vi "SubVI Tester.vi"() -> ()   [LabVIEW 2012]
uses:
  weather data.ctl
panel:
  in  "Max Windspeed":dbl
  in  "Current Windspeed":dbl
  in  "Weather Data In":T1={"Current Temperature"=0.0, "Max Temperature"=0.0, "Min Temperature"=0.0, "Warning Text"="", "Warning?"=FALSE, "Enum"=enum."Fahrenheit", "Current Windspeed"=0.0, "Max Windspeed"=0.0, "Windspeed Warning?"=FALSE, "Windspeed Warning Text"="No Warning"}
  out "Weather Data out":T1={"Current Temperature"=0.0, "Max Temperature"=0.0, "Min Temperature"=0.0, "Warning Text"="", "Warning?"=FALSE, "Enum"=enum."Fahrenheit", "Current Windspeed"=0.0, "Max Windspeed"=0.0, "Windspeed Warning?"=FALSE, "Windspeed Warning Text"="No Warning"}
  in  "Min Temperature":dbl=10.0
  in  "Max Temperature":dbl=30.0
  in  "Stop":bool
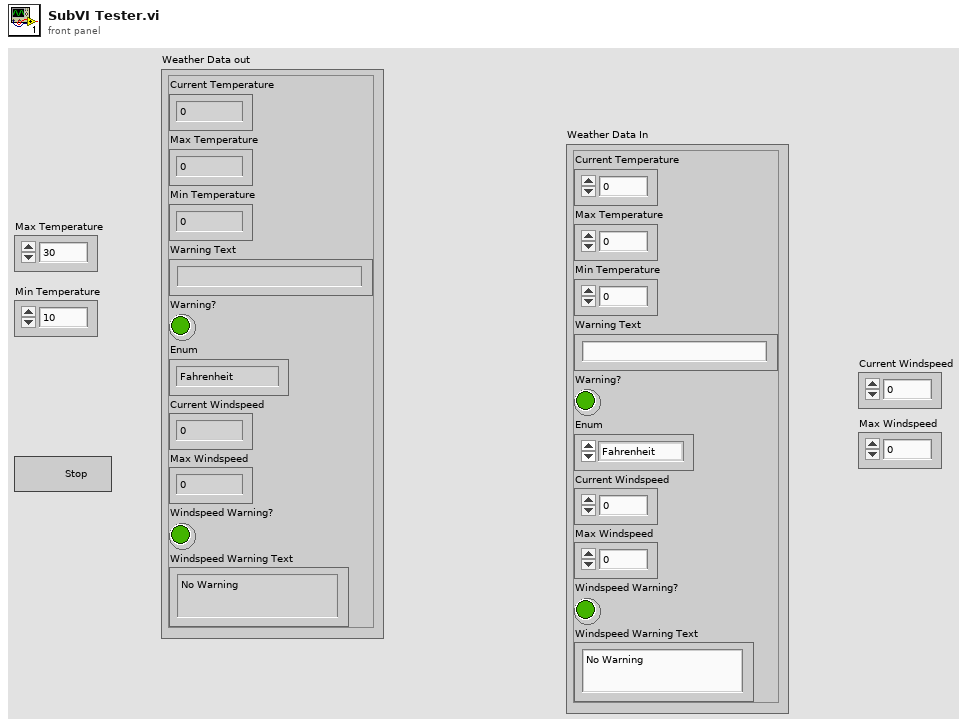
[diagram p1: front panel]
types:
  T1 = typedef "weather data.ctl" = cluster{"Current Temperature":dbl, "Max Temperature":dbl, "Min Temperature":dbl, "Warning Text":string, "Warning?":bool, "Enum":enum16{"Fahrenheit", "Celcius"}, "Current Windspeed":dbl, "Max Windspeed":dbl, "Windspeed Warning?":bool, "Windspeed Warning Text":string}
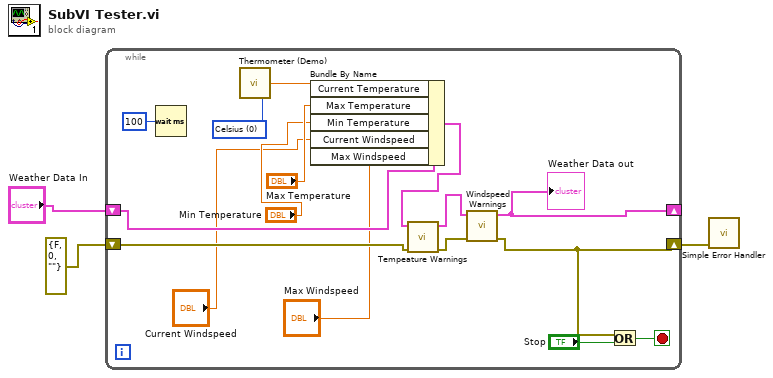
[diagram p0: block diagram]
diagram:
  n1 = while {
    shift-right: [w9] -> w3
    shift-left: errorcluster {"status"=FALSE, "code"=0, "source"=""} ("error in") -> [w16]
    shift-right: [w6] -> _
    shift-left: "Weather Data In" -> [w12]
    stop <- w17 stop-if-true
    w10 = u16 0 items=["Celsius", "Fahrenheit"] ("Units (0: Celsius)")
    n2 = Wait (ms)(milliseconds to wait=u32 100) -> ()  [unwired: 1 out]
    n3 = call "Thermometer (Demo).vi"("Units (0: Celsius)"=w10) -> ("Temperature Value"=w15:dbl)
    n4 = Bundle By Name "Bundle By Name"(cluster=w12, "Current Temperature"=w15, "Max Temperature"="Max Temperature", "Min Temperature"="Min Temperature", "Current Windspeed"="Current Windspeed", "Max Windspeed"="Max Windspeed") -> (w11:T1)
    n5 = call "Tempeature Warnings.vi"("error in (no error)"=w16, "Weather Data In"=w11) -> ("error out"=w8:errorcluster, "Weather Data out"=w7:T1)  [unwired: 8 in]
    n6 = call "Windspeed Warnings.vi"("error in"=w8, "Weather Data In"=w7) -> ("error out"=w9:errorcluster, "Weather Data Out"=w6:T1)  [unwired: 8 in]
    "Weather Data out" <- w6
    n7 = Or(x=w9, y="Stop") -> (x .or. y?=w17:bool)
  }
  n8 = call <vilib>:"Simple Error Handler.vi"("error in (no error)"=w3) -> ()  [unwired: 4 in, 5 out]
